vi "GlobalCommandFinishedFlag.vi"() -> ()   [LabVIEW 2020]
panel:
  in  "CommandFinishedFlag":bool
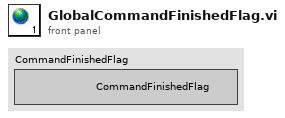
[diagram p1: front panel]
diagram:
